vi "DAQmx.44xx.Get Terminal Coupling.vi"(8 "error in (no error)":errorcluster, 9 "Channel in":tag, 11 "Coupling in":T1=10045 items=[""=0, "AC"=10045, "DC"=10050, "GND"=10066]) -> (0 "error out":errorcluster, 3 "AI.Coupling":i32(ring)=10045 items=["AC"=10045, "DC"=10050, "GND"=10066])   [LabVIEW 2019, in "DAQmx.lvclass"]
uses:
  DAQmx.lvclass
  typedefs/DAQ.Config.AI.Coupling--enum.ctl
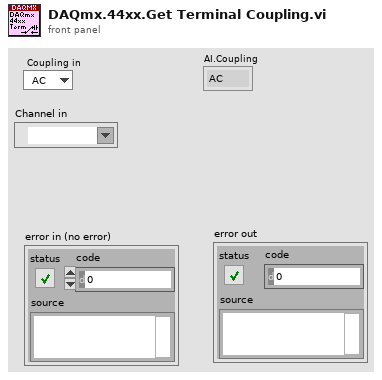
[diagram p1: front panel]
types:
  T1 = typedef "DAQmx.lvclass/DAQ.Config.AI.Coupling--enum.ctl" = u16
  T2 = typedef "DAQmx.lvclass/DAQ.Config.Device Type--enum.ctl" = enum16{"None", "USB-4431", "PXI-446x"}
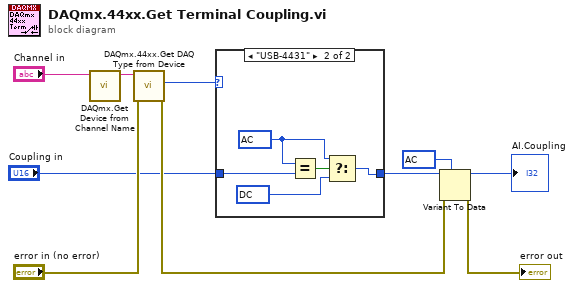
[diagram p0: block diagram]
diagram:
  w7 = 10045 items=["AC"=10045, "DC"=10050, "GND"=10066] ("AI.Coupling")
  n1 = call "DAQmx.Get Device from Channel Name.vi"("Channel"="Channel in") -> ("Device"=w10:tag)  [unwired: 10 in]
  n2 = call "DAQmx.44xx.Get DAQ Type from Device.vi"("error in (no error)"="error in (no error)", "DAQmx Device Name"=w10) -> ("error out"=w5:errorcluster, "DAQ Type"=w3:T2)  [unwired: 7 in, 1 out]
  n3 = case shown="\"USB-4431\"" w3 {
    tunnel: "Coupling in" -> [w11 w16]
    tunnel: [w11 w14] -> w1
    frame Default {
    }
    frame "USB-4431" {
      w13 = T1 10050 items=[""=0, "AC"=10045, "DC"=10050, "GND"=10066] ("Coupling in")
      w12 = T1 10045 items=[""=0, "AC"=10045, "DC"=10050, "GND"=10066] ("Coupling in")
      n4 = Equal?(x=w12, y=w16) -> (x = y?=w15:bool)
      n5 = Select(t=w12, s=w15, f=w13) -> (s? t:f=w14:T1)
    }
  }
  n6 = Variant To Data(error in=w5, type=w7, Variant=w1) -> (data=→"AI.Coupling":i32, error out=→"error out":errorcluster)
